vi "Full Density Matrix - Read.vi"(7 "QuWire in":refnum<class "QuWire.lvclass">) -> (8 "Full Density Matrix":cdb[][](array[numeric]))   [LabVIEW 2020]
uses:
  QuSim/QuWire/QuWire.lvclass
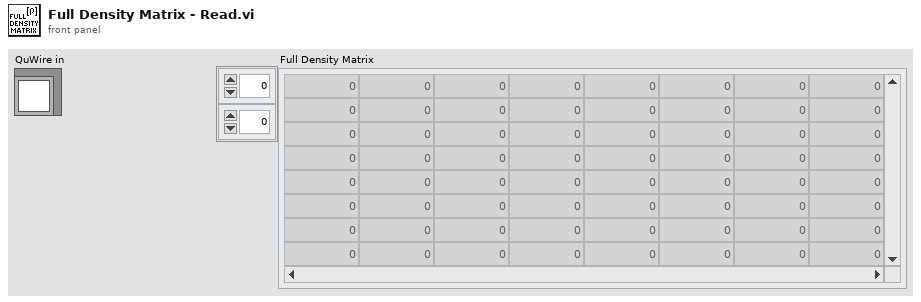
[diagram p1: front panel]
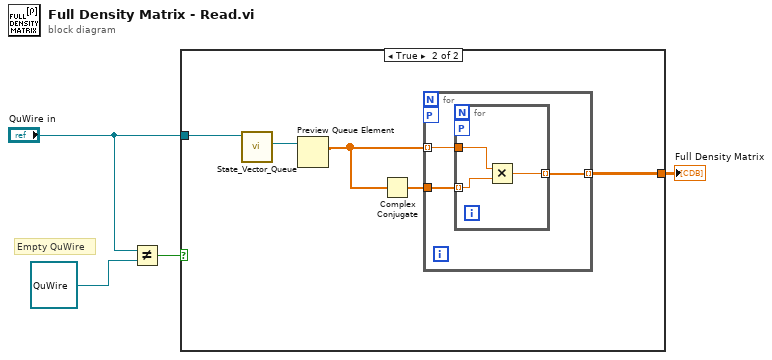
[diagram p0: block diagram]
diagram:
  # "Empty QuWire"
  n1 = Not Equal?(x="QuWire in", y=refnum<class "QuWire.lvclass"> refnum ("QuWire in")) -> (x != y?=w2:bool)
  n2 = case shown="True" w2 {
    tunnel: "QuWire in" -> [_ w8]
    tunnel: [_ w5] -> w1
    frame False {
    }
    frame True {
      n3 = call "State_Vector_Queue.vi"("QuWire in"=w8) -> ("State Vector Queue"=w9:refnum<queue>)  [unwired: 8 in, 2 out]
      n4 = Preview Queue Element(queue=w9) -> (element=w6:cdb[])  [unwired: 2 in, 3 out]
      n5 = Complex Conjugate(1:w6) -> (0:w7:cdb[])
      n6 = for {
        tunnel: w6 -> [w11] mode=indexing
        tunnel: w7 -> [w12]
        tunnel: [w10] -> w5 mode=indexing
        workers-P: _ -> [_]
        n7 = for {
          tunnel: w12 -> [w14] mode=indexing
          tunnel: w11 -> [w15]
          tunnel: [w13] -> w10 mode=indexing
          workers-P: _ -> [_]
          n8 = Multiply(x=w15, y=w14) -> (x*y=w13:cdb)
        }
      }
    }
  }
  "Full Density Matrix" <- w1
